vi "LWXPS_PositionerCorrectorPIDFFVelocitySet.vi"(0 "Proportional gain":dbl, 1 "Integral gain":dbl, 2 "Derivative gain":dbl, 3 "Integral saturation value":dbl, 4 "Integration time":dbl, 5 "Derivative filter cut off frequency":dbl, 6 "Proportional gain multiplier":dbl, 7 "Integral gain multiplier":dbl, 8 "Closed Loop Status":bool, 9 "Derivative gain multiplier":dbl, 10 "Positioner Name":string, 11 "Form coefficient":dbl, 12 "XPS Reference IN":refnum<k24>, 13 "Feed forward velocity":dbl, 15 "LabVIEW error IN":errorcluster) -> (20 "XPS Reference OUT":refnum<k24>, 22 "Returned error code":i32, 25 "XPS Error String":string, 27 "LabVIEW error OUT":errorcluster)   [LabVIEW 2014]
uses:
  D:/XPSQ8_LabView_Library/Development/Source/Dll/Newport.XPS.CommandInterface.dll
  Dll/Newport.XPS.CommandInterface.dll
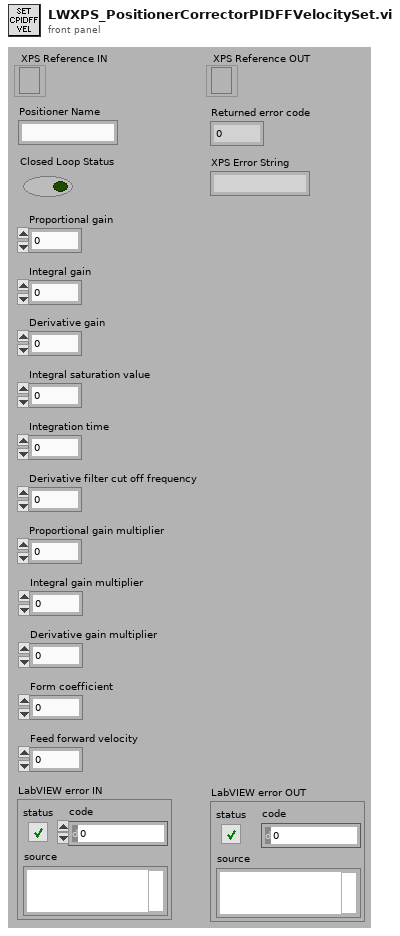
[diagram p1: front panel]
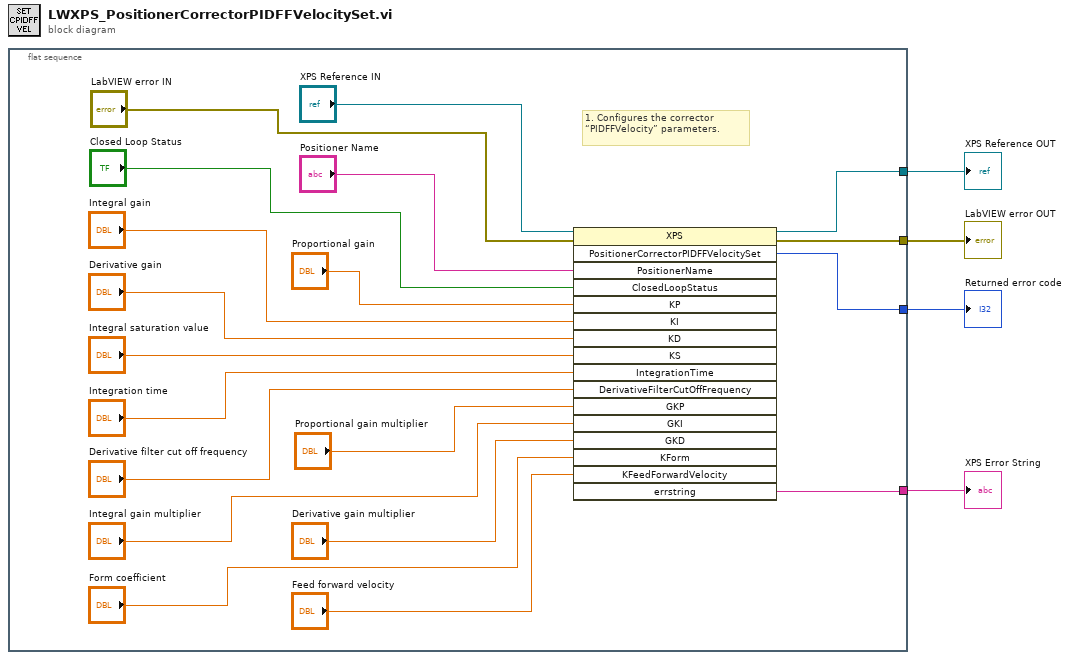
[diagram p0: block diagram]
diagram:
  n1 = flat-sequence {
    tunnel: [w9] -> w4
    tunnel: [w22] -> w3
    tunnel: [w21] -> w2
    tunnel: [w8] -> w1
    frame #0 {
      # "1. Configures the corrector “PIDFFVelocity” parameters."
      n2 = invoke class="XPS" method="PositionerCorrectorPIDFFVelocitySet"(reference="XPS Reference IN", error in="LabVIEW error IN", "PositionerName"="Positioner Name", "ClosedLoopStatus"="Closed Loop Status", "KP"="Proportional gain", "KI"="Integral gain", "KD"="Derivative gain", "KS"="Integral saturation value", "IntegrationTime"="Integration time", "DerivativeFilterCutOffFrequency"="Derivative filter cut off frequency", "GKP"="Proportional gain multiplier", "GKI"="Integral gain multiplier", "GKD"="Derivative gain multiplier", "KForm"="Form coefficient", "KFeedForwardVelocity"="Feed forward velocity") -> (reference out=w9:refnum<k24>, error out=w22:errorcluster, "PositionerCorrectorPIDFFVelocitySet"=w21:i32, "errstring"=w8:string)  [unwired: 2 in, 13 out]
    }
  }
  "XPS Error String" <- w1
  "XPS Reference OUT" <- w4
  "LabVIEW error OUT" <- w3
  "Returned error code" <- w2
